vi "python analysis testing.vi"() -> ()   [LabVIEW 2020]
uses:
  <vilib>/vision/Image Controls.llb/IMAQ Image.ctl
panel:
  out "return value":dbl[](array[numeric])
  out "error out":errorcluster
  in  "Image Type":T1 items=["Grayscale (U8)", "Grayscale (I16)", "Grayscale (SGL)", "Complex (CSG)", "RGB (U32)", "HSL (U32)", "RGB (U64)", "Grayscale (U16)"]
  out "Image":T2(plugin-control)
  out "Image Out":T2
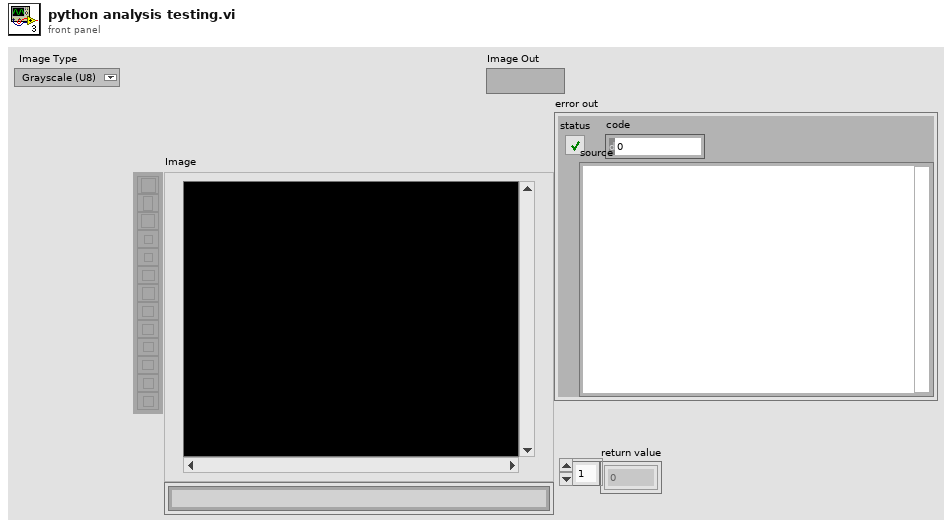
[diagram p1: front panel]
types:
  T1 = typedef "Image Type" = u32
  T2 = typedef "IMAQ Image.ctl" = refnum<image>
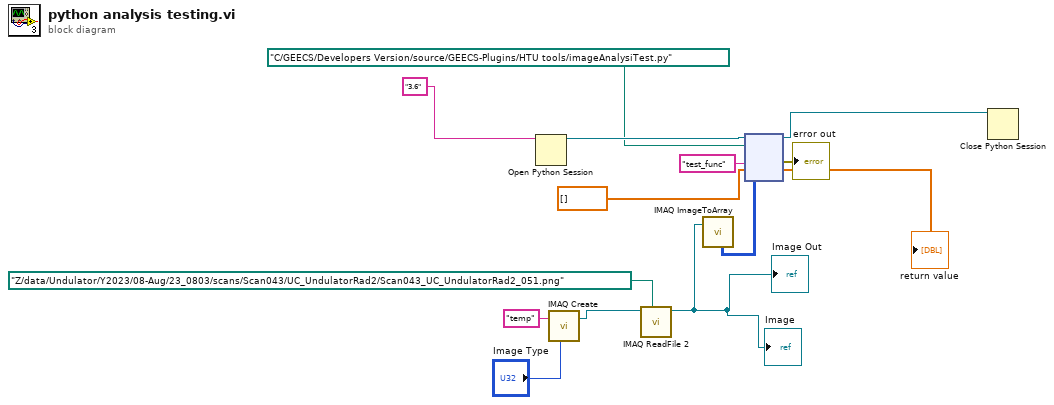
[diagram p0: block diagram]
diagram:
  n1 = Open Python Session(python version="3.6" ("Python version")) -> (session out=w9:refnum<k35>)  [unwired: 2 in, 1 out]
  n2 = call "IMAQ Create"("Image Name"="temp", "Image Type"="Image Type") -> ("New Image"=w13:T2)  [unwired: 3 in, 1 out]
  n3 = call "IMAQ ReadFile 2"("File Path"=path "Z:/data/Undulator/Y2023/08-Aug/23_0803/scans/Scan043/UC_UndulatorRad2/Scan043_UC_UndulatorRad2_051.png", "Image"=w13) -> ("Image Out"=w10:T2)  [unwired: 5 in, 4 out]
  "Image Out" <- w10
  "Image" <- w10
  n4 = call "IMAQ ImageToArray"("Image"=w10) -> ("Image Pixels (U16)"=w2:u16[][])  [unwired: 3 in, 4 out]
  n5 = node(w9, path "C:/GEECS/Developers Version/source/GEECS-Plugins/HTU tools/imageAnalysiTest.py" ("module path"), "test_func" ("function name"), dbl[] [], w2) -> (w8:refnum<k35>, →"error out":errorcluster, →"return value":dbl[])  [unwired: 2 in, 2 out]
  n6 = Close Python Session(session in=w8) -> ()  [unwired: 1 in, 1 out]
